vi "EditorSub relayoutListbox.vi"(7 "function":enum16{"init", "run"}(ring), 8 "error in (no error)":errorcluster, 9 "listboxPaneRefnum":refnum<vi>, 11 "listboxRefnum":refnum<vi>) -> (0 "error out":errorcluster)   [LabVIEW 2018]
uses:
  <vilib>/Utility/miscctls.llb/LVRowAndColumnTypeDef.ctl
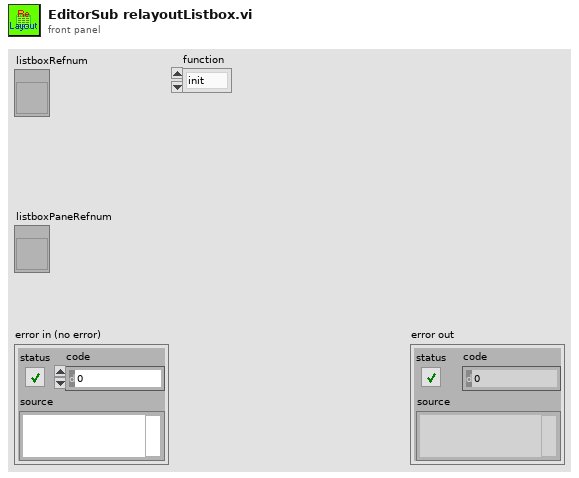
[diagram p1: front panel]
types:
  T1 = typedef "LVRowAndColumnTypeDef.ctl" = cluster{"Row":i32, "Column":i32}
  T2 = typedef "LVBoundsTypeDef.ctl" = cluster{"Width":u32, "Height":u32}
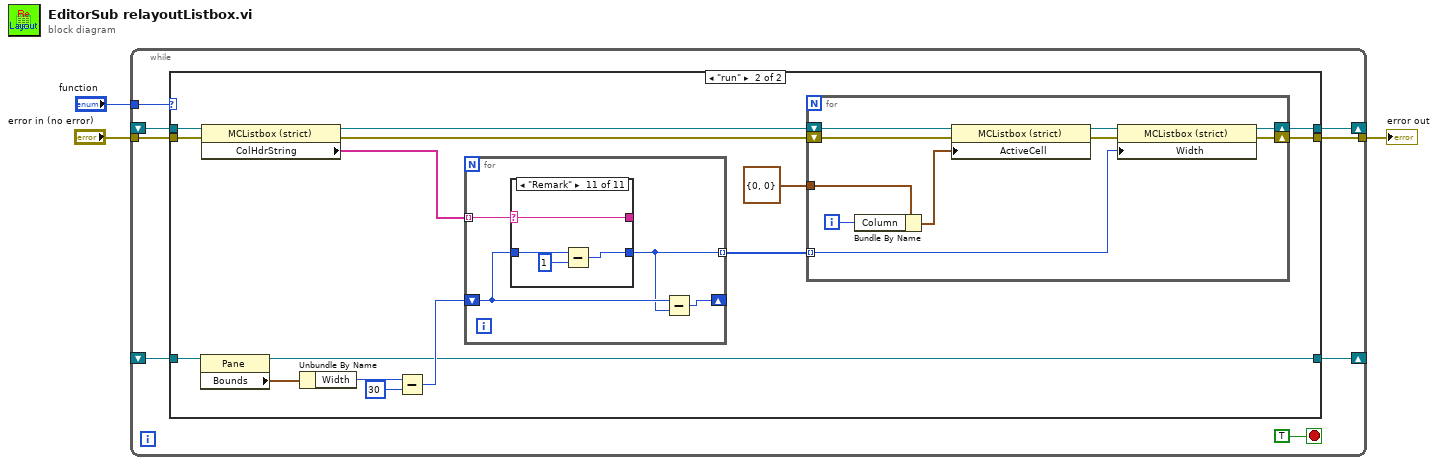
[diagram p0: block diagram]
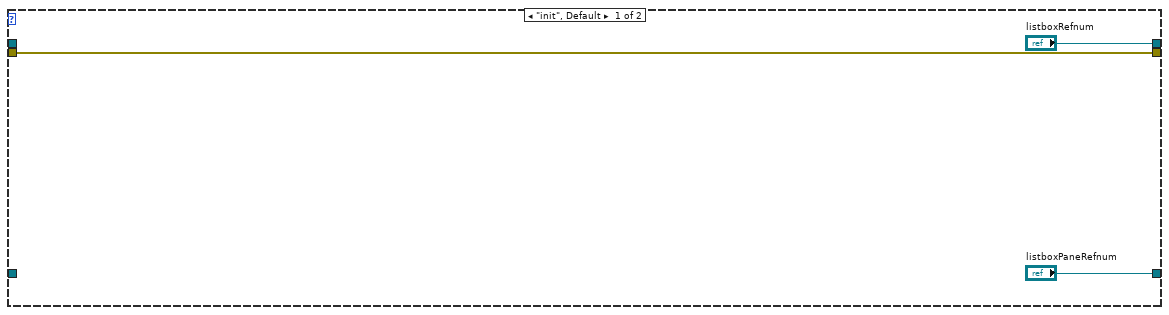
[diagram p2: hidden frame]
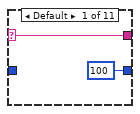
[diagram p3: hidden frame]
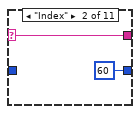
[diagram p4: hidden frame]
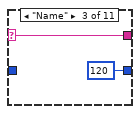
[diagram p5: hidden frame]
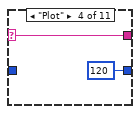
[diagram p6: hidden frame]
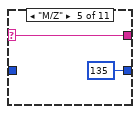
[diagram p7: hidden frame]
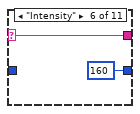
[diagram p8: hidden frame]
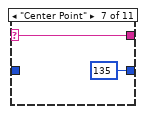
[diagram p9: hidden frame]
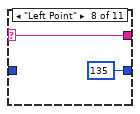
[diagram p10: hidden frame]
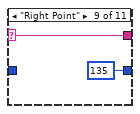
[diagram p11: hidden frame]
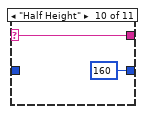
[diagram p12: hidden frame]
diagram:
  n1 = while {
    tunnel: "function" -> [w11]
    shift-right: [w10] -> _
    shift-left: _ -> [w8]
    shift-right: [w9] -> _
    shift-left: _ -> [w7]
    tunnel: "error in (no error)" -> [w5]
    tunnel: [w4] -> w1
    stop <- TRUE stop-if-true
    n2 = case shown="\"run\"" w11 {
      tunnel: ["listboxRefnum" w17] -> w10
      tunnel: ["listboxPaneRefnum" w22] -> w9
      tunnel: w8 -> [_ w29]
      tunnel: w7 -> [_ w24]
      tunnel: w5 -> [w12 w16]
      tunnel: [w12 w15] -> w4
      frame "init", Default {
      }
      frame "run" {
        n3 = property class="Pane"(reference=w24) -> (reference out=w22:refnum<vi>, "Bounds"=w27:T2)  [unwired: 1 in, 1 out]
        n4 = property class="MCListbox (strict)"(reference=w29, error in=w16) -> (reference out=w21:refnum<vi>, error out=w20:errorcluster, "ColHdrString"=w28:string[])
        n5 = Unbundle By Name(w27) -> ("Width"=w26:u32)
        n6 = Subtract(x=w26, y=u32 30) -> (x-y=w23:u32)
        n7 = for {
          tunnel: w28 -> [w43] mode=indexing
          shift-right: [w42] -> _
          shift-left: w23 -> [w41]
          tunnel: [w40] -> w19 mode=indexing
          n8 = case shown="\"Remark\"" w43 {
            selector: w43 -> [w45 w47 w49 w51 w52 w54 w56 w58 w60 w62 w67]
            tunnel: [u32 100 ("Width") u32 60 ("Width") u32 120 ("Width") u32 120 ("Width") u32 135 ("Width") u32 160 ("Width") u32 135 ("Width") u32 135 ("Width") u32 135 ("Width") u32 160 ("Width") w65] -> w40
            tunnel: [w45 w47 w49 w51 w52 w54 w56 w58 w60 w62 w67] -> _
            tunnel: w41 -> [_ _ _ _ _ _ _ _ _ _ w66]
            frame Default {
            }
            frame "Index" {
            }
            frame "Name" {
            }
            frame "Plot" {
            }
            frame "M/Z" {
            }
            frame "Intensity" {
            }
            frame "Center Point" {
            }
            frame "Left Point" {
            }
            frame "Right Point" {
            }
            frame "Half Height" {
            }
            frame "Remark" {
              n9 = Subtract(x=w66, y=u32 1) -> (x-y=w65:u32)
            }
          }
          n10 = Subtract(x=w41, y=w40) -> (x-y=w42:u32)
        }
        n11 = for {
          tunnel: w19 -> [w32] mode=indexing
          tunnel: T1 {"Row"=0, "Column"=0} ("Active Cell:Active Cell") -> [w35]
          shift-right: [w31] -> w17
          shift-left: w21 -> [w39]
          shift-right: [w30] -> w15
          shift-left: w20 -> [w38]
          i -> [w34]
          n12 = Bundle By Name(cluster=w35, "Column"=w34) -> (w33:T1)
          n13 = property class="MCListbox (strict)"(reference=w39, error in=w38, "ActiveCell"=w33) -> (reference out=w37:refnum<vi>, error out=w36:errorcluster)
          n14 = property class="MCListbox (strict)"(reference=w37, error in=w36, "Width"=w32) -> (reference out=w31:refnum<vi>, error out=w30:errorcluster)
        }
      }
    }
  }
  "error out" <- w1
